vi "Barcode v1.vi"(1 "Board Repair Info":T1, 5 "Tbl Refnum":refnum<vi>, 11 "Barcode In":string) -> (2 "Length":u32, 3 "Barcode":string)   [LabVIEW 2018]
uses:
  Ctl/Repair Data.ctl
  <vilib>/Utility/miscctls.llb/LVSelectionTypeDef.ctl
  <vilib>/Utility/config.llb/Read Key (U32).vi
  <vilib>/Utility/config.llb/Read Key (String).vi
  <vilib>/Utility/config.llb/NI_LVConfig.lvlib
panel:
  out "Exit":bool
  out "Default":string
  out "Mask":string
  out "Ofset":u32
  out "file or folder exists?":bool
  in  "stop":bool
  in  "Save Data":bool
  out "Key Focus":bool
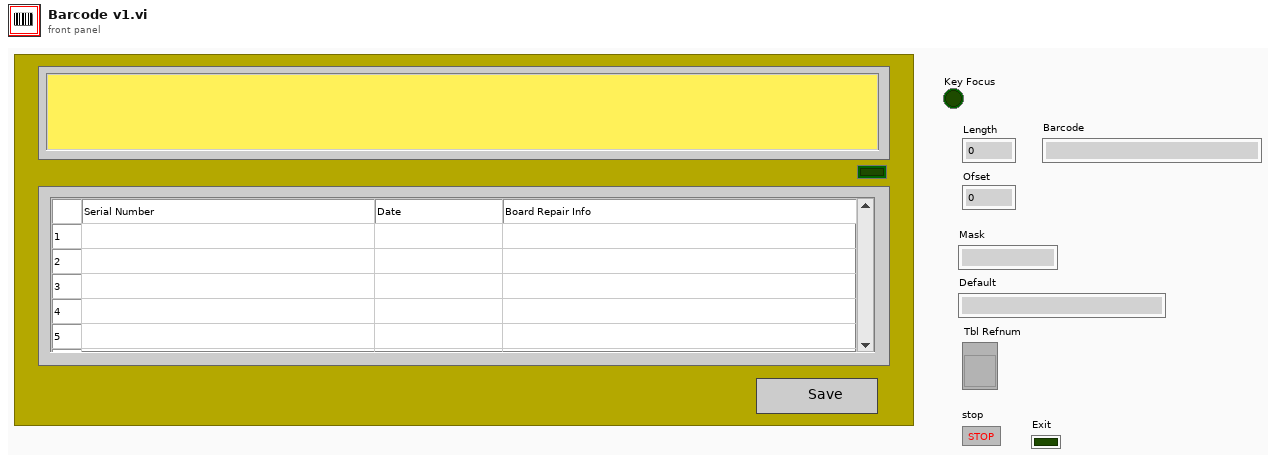
[diagram p1: front panel]
types:
  T1 = typedef "Repair Data.ctl" = string[][]
  T2 = enum32{"Invalid", "Standard", "Closed", "Hidden", "Minimized", "Maximized"}
  T3 = enum32{"Invalid", "Default", "Floating", "Floating/Auto-Hide", "Modal"}
  T4 = typedef "LVSelectionTypeDef.ctl" = cluster{"Selection Start":u32, "Selection End":u32}
  T5 = typedef "NI_LVConfig.lvlib/Config Data RefNum.ctl" = refnum<k1>
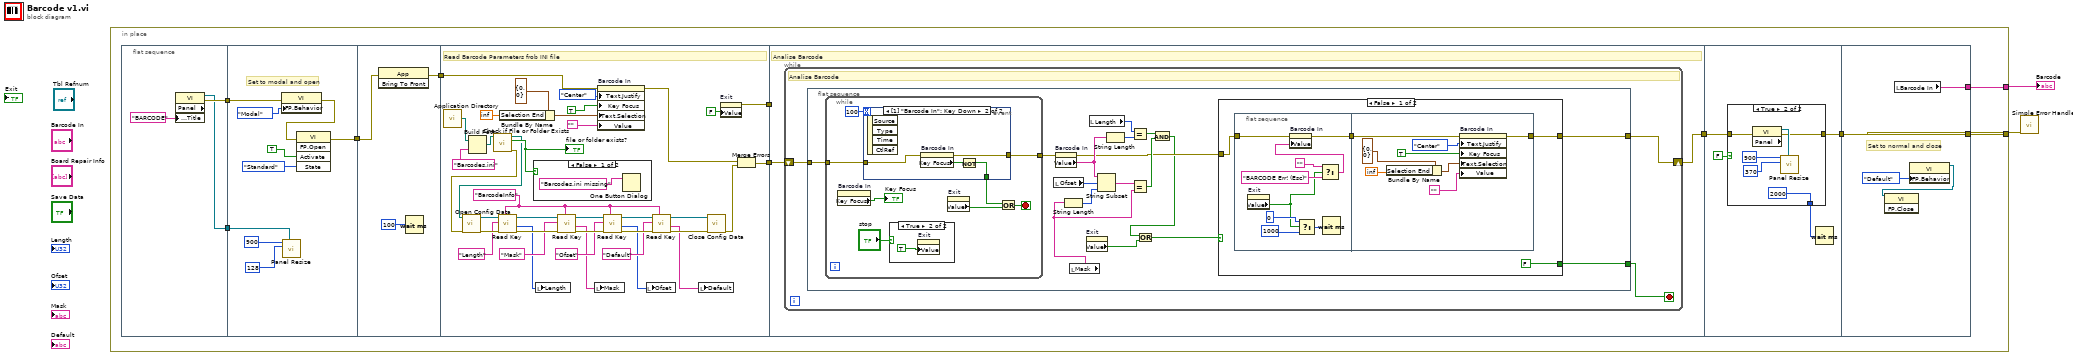
[diagram p0: block diagram]
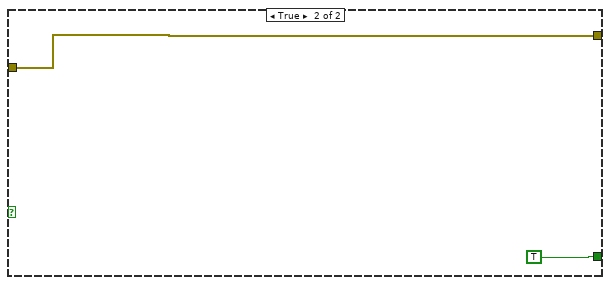
[diagram p3: hidden frame]
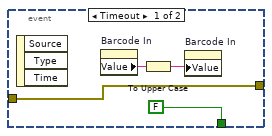
[diagram p5: hidden frame]
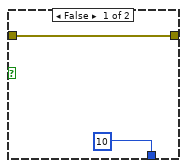
[diagram p6: hidden frame]
diagram:
  n1 = in-place {
    in-place-border: [w6] -> w2
    in-place-border: [w5] -> w1
    n2 = flat-sequence {
      tunnel: [w14] -> w12
      tunnel: [w13] -> w11
      tunnel: [w21] -> w10
      tunnel: w12 -> [w20]
      tunnel: w11 -> [w18]
      tunnel: [w27] -> w9
      tunnel: w10 -> [w25]
      tunnel: w9 -> [w30]
      tunnel: [w41] -> w8
      tunnel: [w28] -> w3
      tunnel: w8 -> [w67]
      tunnel: [w66] -> w4
      tunnel: w3 -> [_]
      tunnel: [w130] -> w7
      tunnel: w4 -> [w131]
      tunnel: [w142] -> w6
      tunnel: w7 -> [w142]
      tunnel: [w141] -> w5
      frame #0 {
        n3 = property class="VI" props=["Panel", "Front Panel.Title"]("Front Panel.Title"="BARCODE" ("Front Panel Window:Title")) -> (reference out=w13:refnum<vi>, error out=w14:errorcluster)  [unwired: 2 in, 1 out]
      }
      frame #1 {
        # "Set to modal and open"
        n4 = property class="VI"(error in=w20, "FP.Behavior"=T3."Modal" ("Front Panel Window:Behavior")) -> (error out=w24:errorcluster)  [unwired: 1 in, 1 out]
        n5 = call "Panel Resize.vi"("Width"=i16 900, "Height"=i16 128, "reference"=w18) -> ()  [unwired: 7 in, 1 out]
        n6 = invoke class="VI" method="FP.Open"(error in=w24, "Activate"=TRUE ("Activate?"), "State"=T2."Standard") -> (error out=w21:errorcluster)  [unwired: 2 in, 4 out]
      }
      frame #2 {
        n7 = invoke class="App" method="Bring To Front"(error in=w25) -> (error out=w27:errorcluster)  [unwired: 2 in, 2 out]
        n8 = Wait (ms)(milliseconds to wait=u32 100) -> ()  [unwired: 1 out]
      }
      frame #3 {
        w49 = "BarcodeInfo"
        # "Read Barcode Parameters frob INI file"
        n9 = call <vilib>:"Application Directory.vi"() -> ("Application Directory"=w57:path)
        n10 = Build Path(base path=w57, name or relative path="Barcodes.ini") -> (appended path=w56:path)
        n11 = call <vilib>:"Check if File or Folder Exists.vi"("path"=w56) -> ("error out"=w53:errorcluster, "file or folder exists?"=w55:bool, "dup path"=w54:path)  [unwired: 8 in]
        "file or folder exists?" <- w55
        n12 = call <vilib>:"Open Config Data.vi"("error in (no error)"=w53, "configuration file path"=w54) -> ("error out"=w45:errorcluster, "refnum"=w52:T5)  [unwired: 7 in, 1 out]
        n13 = call-poly <vilib>:"Read Key.vi"("section"=w49, "error in (no error)"=w45, "key"="Length", "refnum"=w52) -> ("error out"=w46:errorcluster, "value"=w34:u32, "refnum out"=w51:T5)  [unwired: 4 in, 1 out]
        n14 = Bundle By Name(cluster=T4 {"Selection Start"=0, "Selection End"=0} ("Text.Selection"), "Selection End"=inf) -> (w61:T4)
        n15 = case shown="False" w55 {
          frame False {
            n16 = One Button Dialog(message="Barcodes.ini missing") -> ()  [unwired: 1 in, 1 out]
          }
          frame True {
          }
        }
        n17 = local write "Length"(w34) -> ()
        n18 = call-poly <vilib>:"Read Key.vi"("section"=w49, "error in (no error)"=w46, "key"="Mask", "refnum"=w51) -> ("error out"=w47:errorcluster, "value"=w32:string, "refnum out"=w50:T5)  [unwired: 4 in, 1 out]
        n19 = local write "Mask"(w32) -> ()
        n20 = property on="Barcode In" class="Str"(error in=w30, "Text.Justify"=enum16{"Left", "Center", "Right"}."Center" ("Text.Justification"), "Key Focus"=TRUE, "Text.Selection"=w61, "Value"="") -> (error out=w40:errorcluster)  [unwired: 1 in, 1 out]
        n21 = call-poly <vilib>:"Read Key.vi"("section"=w49, "error in (no error)"=w47, "key"="Ofset", "refnum"=w50) -> ("error out"=w48:errorcluster, "value"=w33:u32, "refnum out"=w42:T5)  [unwired: 4 in, 1 out]
        n22 = local write "Ofset"(w33) -> ()
        n23 = call-poly <vilib>:"Read Key.vi"("section"=w49, "error in (no error)"=w48, "key"="Default", "refnum"=w42) -> ("error out"=w44:errorcluster, "value"=w31:string, "refnum out"=w43:T5)  [unwired: 4 in, 1 out]
        n24 = local write "Default"(w31) -> ()
        n25 = call <vilib>:"Close Config Data.vi"("error in (no error)"=w44, "refnum"=w43) -> ("error out"=w39:errorcluster)  [unwired: 8 in, 1 out]
        n26 = property on="Exit" class="Bool (strict)"("Value"=FALSE ("Exit")) -> (error out=w28:errorcluster)  [unwired: 2 in, 1 out]
        n27 = Merge Errors(w40, w39) -> (w41:errorcluster)
      }
      frame #4 {
        # "Analise Barcode"
        n28 = while {
          shift-right: [w68] -> w66
          shift-left: w67 -> [w70]
          stop <- w69 stop-if-true
          # "Analise Barcode"
          n29 = flat-sequence {
            tunnel: [w75] -> w69
            tunnel: [w74] -> w68
            tunnel: w70 -> [w87]
            frame #0 {
              n30 = while {
                tunnel: w87 -> [w115]
                tunnel: [w116] -> w86
                stop <- w114 stop-if-true
                n31 = property on="Barcode In" class="Str"() -> ("Key Focus"=→"Key Focus":bool)  [unwired: 2 in, 2 out]
                n32 = event shown="[1] \"Barcode In\": Key Down" {
                  selector: _ -> [_ _]
                  dyn-events: _ -> [_ _]
                  timeout: 100 -> [_ _]
                  tunnel: [FALSE w126] -> w113
                  tunnel: w115 -> [w120 w125]
                  tunnel: [w120 w124] -> w116
                  event Timeout {
                    n33 = event-data() -> ()  [unwired: 1 in, 3 out]
                    n34 = property on="Barcode In" class="Str"() -> ("Value"=w123:string)  [unwired: 2 in, 2 out]
                    n35 = To Upper Case(1:w123) -> (0:w122:string)
                    n36 = property on="Barcode In" class="Str"("Value"=w122) -> ()  [unwired: 2 in, 2 out]
                  }
                  event "Barcode In": Key Down {
                    n37 = event-data() -> ()  [unwired: 1 in, 4 out]
                    n38 = property on="Barcode In" class="Str"(error in=w125) -> (error out=w124:errorcluster, "Key Focus"=w127:bool)  [unwired: 1 in, 1 out]
                    n39 = Not(x=w127) -> (.not. x?=w126:bool)
                  }
                }
                n40 = case shown="True" "stop" {
                  frame False {
                  }
                  frame True {
                    n41 = property on="Exit" class="Bool (strict)"("Value"=TRUE ("Exit")) -> ()  [unwired: 2 in, 2 out]
                  }
                }
                n42 = property on="Exit" class="Bool (strict)"() -> ("Value"=w111:bool)  [unwired: 2 in, 2 out]
                n43 = Or(x=w113, y=w111) -> (x .or. y?=w114:bool)
              }
              n44 = local read "Ofset"() -> (w82:u32)
              n45 = property on="Barcode In" class="Str"(error in=w86) -> (error out=w76:errorcluster, "Value"=w83:string)  [unwired: 1 in, 1 out]
              n46 = local read "Mask"() -> (w78:string)
              n47 = String Length(string=w78) -> (length=w77:i32)
              n48 = property on="Exit" class="Bool (strict)"() -> ("Value"=w73:bool)  [unwired: 2 in, 2 out]
              n49 = local read "Length"() -> (w84:u32)
              n50 = String Subset(string=w83, offset (0)=w82, length (rest)=w77) -> (substring=w81:string)
              n51 = String Length(string=w83) -> (length=w85:i32)
              n52 = Equal?(x=w84, y=w85) -> (x = y?=w79:bool)
              n53 = Equal?(x=w81, y=w78) -> (x = y?=w80:bool)
              n54 = And(x=w79, y=w80) -> (x .and. y?=w72:bool)
              n55 = Or(x=w72, y=w73) -> (x .or. y?=w71:bool)
              n56 = case shown="False" w71 {
                tunnel: [FALSE TRUE] -> w75
                tunnel: [w90 w109] -> w74
                tunnel: w76 -> [w88 w109]
                frame False {
                  n57 = flat-sequence {
                    tunnel: [w100] -> w89
                    tunnel: w88 -> [w99]
                    tunnel: [w105] -> w90
                    tunnel: w89 -> [w104]
                    frame #0 {
                      n58 = property on="Exit" class="Bool (strict)"() -> ("Value"=w92:bool)  [unwired: 2 in, 2 out]
                      n59 = Select(t=u32 0 ("milliseconds to wait"), s=w92, f=u32 1000 ("milliseconds to wait")) -> (s? t:f=w95:u32)
                      n60 = Select(t="", s=w92, f="BARCODE Err! (Esc)") -> (s? t:f=w98:string)
                      n61 = property on="Barcode In" class="Str"(error in=w99, "Value"=w98) -> (error out=w100:errorcluster)  [unwired: 1 in, 1 out]
                      n62 = Wait (ms)(milliseconds to wait=w95) -> ()  [unwired: 1 out]
                    }
                    frame #1 {
                      n63 = Bundle By Name(cluster=T4 {"Selection Start"=0, "Selection End"=0} ("Text.Selection"), "Selection End"=inf) -> (w102:T4)
                      n64 = property on="Barcode In" class="Str"(error in=w104, "Text.Justify"=enum16{"Left", "Center", "Right"}."Center" ("Text.Justification"), "Key Focus"=TRUE, "Text.Selection"=w102, "Value"="") -> (error out=w105:errorcluster)  [unwired: 1 in, 1 out]
                    }
                  }
                }
                frame True {
                }
              }
            }
          }
        }
      }
      frame #5 {
        n65 = case shown="True" FALSE {
          tunnel: w131 -> [w133 w136]
          tunnel: [w133 w135] -> w130
          tunnel: [10 u32 2000 ("milliseconds to wait")] -> w128
          frame False {
          }
          frame True {
            n66 = property class="VI" props=["Panel"](error in=w136) -> (reference out=w137:refnum<vi>, error out=w135:errorcluster)  [unwired: 1 in, 1 out]
            n67 = call "Panel Resize.vi"("Width"=i16 900, "Height"=i16 370, "reference"=w137) -> ()  [unwired: 7 in, 1 out]
          }
        }
        n68 = Wait (ms)(milliseconds to wait=w128) -> ()  [unwired: 1 out]
      }
      frame #6 {
        # "Set to normal and close"
        n69 = local read "Barcode In"() -> (w141:string)
        n70 = property class="VI"("FP.Behavior"=T3."Default" ("Front Panel Window:Behavior")) -> (reference out=w140:refnum<vi>)  [unwired: 2 in, 1 out]
        n71 = invoke class="VI" method="FP.Close"(reference=w140) -> ()  [unwired: 2 in, 3 out]
      }
    }
  }
  "Barcode" <- w1
  n72 = call <vilib>:"Simple Error Handler.vi"("error in (no error)"=w2) -> ()  [unwired: 4 in, 5 out]
